vi "ABR3-Compute Corrcoefs.vi"(0 "Level (in)":dbl[](array[numeric]), 5 "Neural":dbl[][](array[numeric]), 7 "dt (us)":dbl, 9 "Threshold Estimation":T1, 11 "error in (no error)":errorcluster) -> (4 "Level (out)":dbl[](array[numeric]), 6 "Corrcoefs":dbl[](array[numeric]), 15 "error out":errorcluster)   [LabVIEW 2020]
uses:
  ABR3-Threshold Estimation Parameters.ctl
  1cd5d013-2a3c-4250-bace-59f0c5ec0f04.vi
  <vilib>/Analysis/baseanly.llb/Mean.vi
  <vilib>/Analysis/baseanly.llb/Mean (DBL).vi
  epl-vi-lib/Utility VIs/Array Manipulation VIs/Array-Dimensions (2D).vi
  <vilib>/gmath/NI_Gmath.lvlib
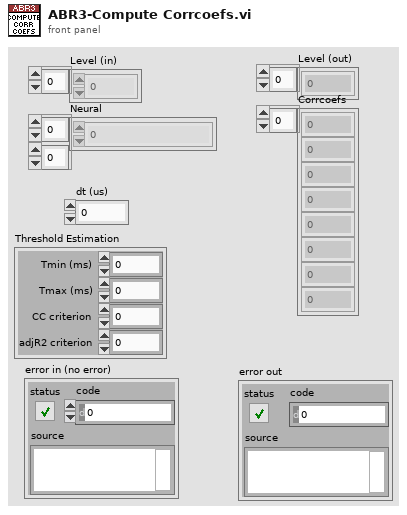
[diagram p1: front panel]
types:
  T1 = typedef "ABR3-Threshold Estimation Parameters.ctl" = cluster{"Tmin (ms)":dbl, "Tmax (ms)":dbl, "CC criterion":dbl, "adjR2 criterion":dbl}
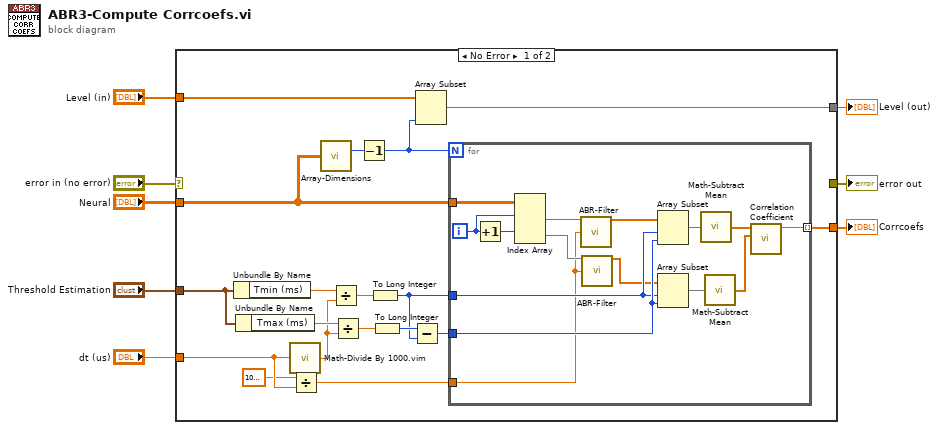
[diagram p0: block diagram]
diagram:
  n1 = case shown="No Error" "error in (no error)" {
    selector: "error in (no error)" -> [_ w42]
    tunnel: "Threshold Estimation" -> [w22 _]
    tunnel: [w16 _] -> w7
    tunnel: [w15 _] -> w8
    tunnel: [_ w42] -> w4
    tunnel: "Level (in)" -> [w14 _]
    tunnel: "Neural" -> [w13 _]
    tunnel: "dt (us)" -> [w11 _]
    frame No Error {
      n2 = Unbundle By Name(w22) -> ("Tmin (ms)"=w26:dbl)
      n3 = Unbundle By Name(w22) -> ("Tmax (ms)"=w24:dbl)
      n4 = call "Math-Divide By 1000.vim"("X"=w11) -> ("1000X"=w21:dbl)
      n5 = Divide(x=1000000.0, y=w11) -> (x/y=w9:dbl)
      n6 = call-poly "Array-Dimensions.vi"("2D Array"=w13) -> ("# rows"=w20:i32)  [unwired: 13 in, 1 out]
      n7 = Divide(x=w26, y=w21) -> (x/y=w25:dbl)
      n8 = Divide(x=w24, y=w21) -> (x/y=w23:dbl)
      n9 = Decrement(x=w20) -> (x-1=w12:i32)
      n10 = To Long Integer(number=w25) -> (32bit integer=w18:i32)
      n11 = To Long Integer(number=w23) -> (32bit integer=w19:i32)
      n12 = Subtract(x=w19, y=w18) -> (x-y=w17:i32)
      n13 = Array Subset(array=w14, length=w12) -> (w15:dbl[])  [unwired: 1 in]
      n14 = for {
        N: w12 -> [_]
        tunnel: w13 -> [w41]
        tunnel: w18 -> [w37]
        tunnel: w17 -> [w38]
        tunnel: [w34] -> w16 mode=indexing
        tunnel: w9 -> [w27]
        i -> [w40]
        n15 = Increment(x=w40) -> (x+1=w39:i32)
        n16 = Index Array(array=w41, index (row) #1=w40, index (row) #2=w39) -> (element #1=w31:dbl[], element #2=w29:dbl[])  [unwired: 2 in]
        n17 = call "ABR-Filter.vi"("ABR raw"=w31, "sampling freq: fs"=w27) -> ("ABR filtered"=w30:dbl[])  [unwired: 12 in, 1 out]
        n18 = call "ABR-Filter.vi"("ABR raw"=w29, "sampling freq: fs"=w27) -> ("ABR filtered"=w28:dbl[])  [unwired: 12 in, 1 out]
        n19 = Array Subset(array=w30, index=w37, length=w38) -> (w36:dbl[])
        n20 = Array Subset(array=w28, index=w37, length=w38) -> (w35:dbl[])
        n21 = call "Math-Subtract Mean.vi"("Y"=w36) -> ("Y - mean(Y)"=w33:dbl[])  [unwired: 4 in]
        n22 = call "Math-Subtract Mean.vi"("Y"=w35) -> ("Y - mean(Y)"=w32:dbl[])  [unwired: 4 in]
        n23 = call <vilib>:"Correlation Coefficient.vi"("Y"=w32, "X"=w33) -> ("correlation coefficient r"=w34:dbl)  [unwired: 8 in, 1 out]
      }
    }
    frame Error {
    }
  }
  "Level (out)" <- w8
  "Corrcoefs" <- w7
  "error out" <- w4
